vi "Canny分割算法.vi"() -> ()   [LabVIEW 2018]
uses:
  <vilib>/Utility/error.llb/DialogType.ctl
  <vilib>/vision/NI_Vision_Development_Module.lvlib
  Dll/Canny_fillhole.dll
panel:
  in  "保存":bool
  out "像素当量单位":string
  out "像素当量":string
  out "是否进行像素标定":bool
  in  "单帧回看":bool
  out "火焰帧数":string
  in  "重新选择":bool
  in  "火焰详细参数":bool
  out "叠加部分":string
  out "单帧部分":string
  out "原图":T1(plugin-control)
  in  "返回主界面":bool
  in  "程序停止":bool
  out "Progress Bar":i32(slide) max=41 scale=-1.0..41.0
  out "单帧火焰":T1(plugin-control)
  out "叠加火焰":T1(plugin-control)
  # "基于Canny算法的炮口火焰分割"
  # "火\n焰\n参\n数"
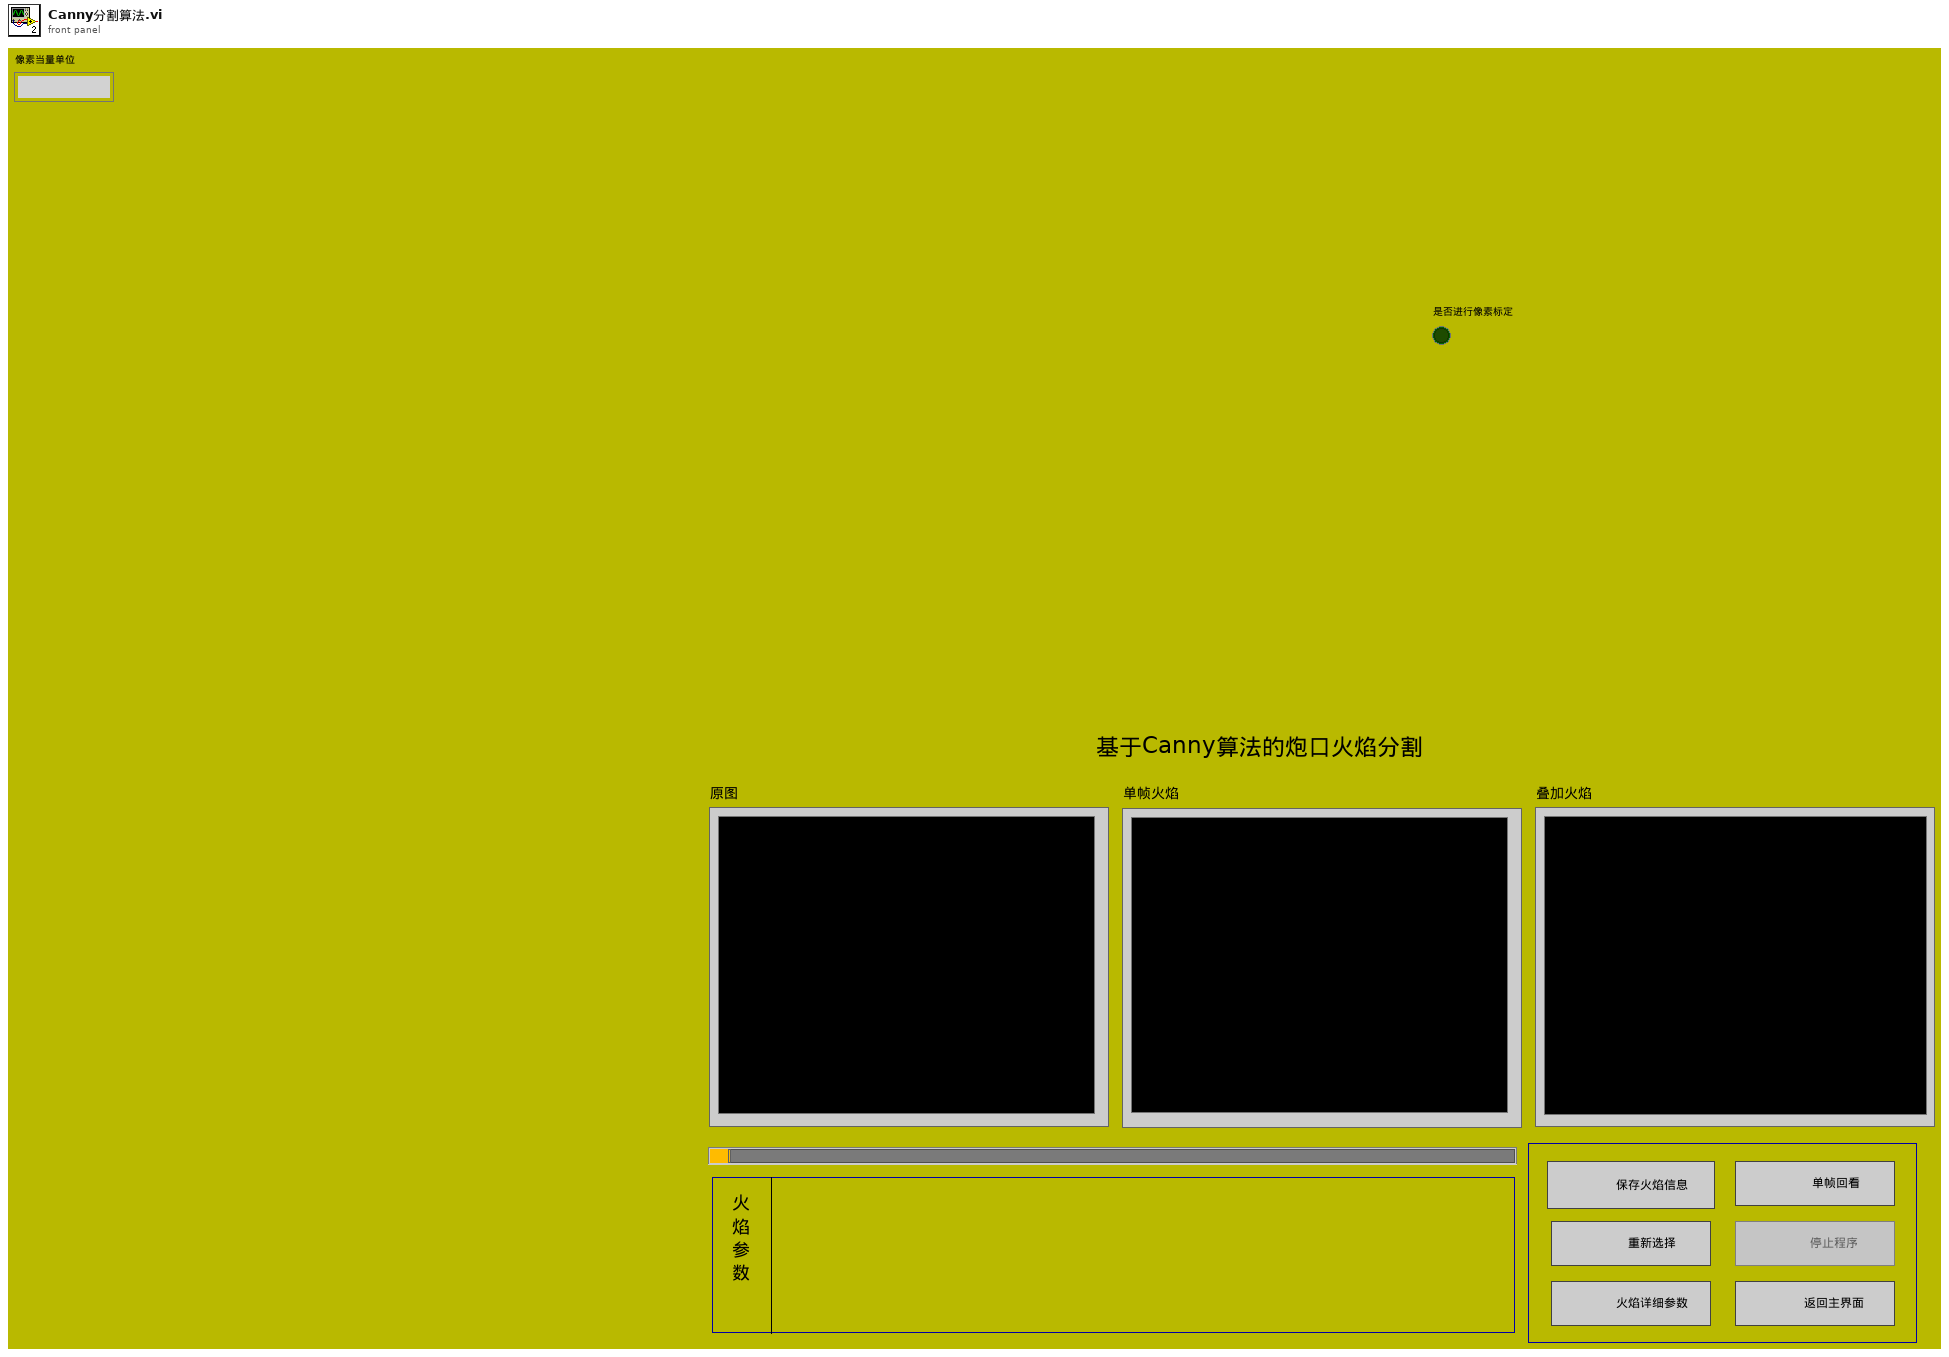
[diagram p1: front panel]
types:
  T1 = typedef "IMAQ Image.ctl" = refnum<image>
  T2 = enum8{"Enabled", "Disabled", "Disabled and Grayed Out"}
  T3 = enum32{"Invalid", "Standard", "Closed", "Hidden", "Minimized", "Maximized"}
  T4 = typedef "DialogType.ctl" = u16
  T5 = typedef "Image Type" = u32
  T6 = typedef "IMAQ AVI2 Refnum.ctl" = refnum<k20>
  T7 = cluster{"Width":u32, "Height":u32, "Frames Per Second":u32, "Codec":string, "Has Data":bool}
  T8 = typedef "ROI Descriptor" = cluster{"Global Rectangle":i32[], "Contours":cluster{"ID":enum32{"External", "Internal"}, "Type":u32, "Coordinates":i32[]}[]}
  T9 = cluster{"Area":dbl, "Number of Holes":dbl, "Bounding Rect":cluster{"Left":dbl, "Top":dbl, "Right":dbl, "Bottom":dbl}, "Center of Mass":cluster{"X":dbl, "Y":dbl}, "Orientation":dbl, "Dimensions":cluster{"Width":dbl, "Height":dbl}}[]
  T10 = cluster{"Particle Reports (Pixels)[0]":cluster{"Area":dbl, "Number of Holes":dbl, "Bounding Rect":cluster{"Left":dbl, "Top":dbl, "Right":dbl, "Bottom":dbl}, "Center of Mass":cluster{"X":dbl, "Y":dbl}, "Orientation":dbl, "Dimensions":cluster{"Width":dbl, "Height":dbl}}, "Particle Reports (Pixels)[1]":cluster{"Area":dbl, "Number of Holes":dbl, "Bounding Rect":cluster{"Left":dbl, "Top":dbl, "Right":dbl, "Bottom":dbl}, "Center of Mass":cluster{"X":dbl, "Y":dbl}, "Orientation":dbl, "Dimensions":cluster{"Width":dbl, "Height":dbl}}, "Particle Reports (Pixels)[2]":cluster{"Area":dbl, "Number of Holes":dbl, "Bounding Rect":cluster{"Left":dbl, "Top":dbl, "Right":dbl, "Bottom":dbl}, "Center of Mass":cluster{"X":dbl, "Y":dbl}, "Orientation":dbl, "Dimensions":cluster{"Width":dbl, "Height":dbl}}, "Particle Reports (Pixels)[3]":cluster{"Area":dbl, "Number of Holes":dbl, "Bounding Rect":cluster{"Left":dbl, "Top":dbl, "Right":dbl, "Bottom":dbl}, "Center of Mass":cluster{"X":dbl, "Y":dbl}, "Orientation":dbl, "Dimensions":cluster{"Width":dbl, "Height":dbl}}, "Particle Reports (Pixels)[4]":cluster{"Area":dbl, "Number of Holes":dbl, "Bounding Rect":cluster{"Left":dbl, "Top":dbl, "Right":dbl, "Bottom":dbl}, "Center of Mass":cluster{"X":dbl, "Y":dbl}, "Orientation":dbl, "Dimensions":cluster{"Width":dbl, "Height":dbl}}, "Particle Reports (Pixels)[5]":cluster{"Area":dbl, "Number of Holes":dbl, "Bounding Rect":cluster{"Left":dbl, "Top":dbl, "Right":dbl, "Bottom":dbl}, "Center of Mass":cluster{"X":dbl, "Y":dbl}, "Orientation":dbl, "Dimensions":cluster{"Width":dbl, "Height":dbl}}, "Particle Reports (Pixels)[6]":cluster{"Area":dbl, "Number of Holes":dbl, "Bounding Rect":cluster{"Left":dbl, "Top":dbl, "Right":dbl, "Bottom":dbl}, "Center of Mass":cluster{"X":dbl, "Y":dbl}, "Orientation":dbl, "Dimensions":cluster{"Width":dbl, "Height":dbl}}, "Particle Reports (Pixels)[7]":cluster{"Area":dbl, "Number of Holes":dbl, "Bounding Rect":cluster{"Left":dbl, "Top":dbl, "Right":dbl, "Bottom":dbl}, "Center of Mass":cluster{"X":dbl, "Y":dbl}, "Orientation":dbl, "Dimensions":cluster{"Width":dbl, "Height":dbl}}, "Particle Reports (Pixels)[8]":cluster{"Area":dbl, "Number of Holes":dbl, "Bounding Rect":cluster{"Left":dbl, "Top":dbl, "Right":dbl, "Bottom":dbl}, "Center of Mass":cluster{"X":dbl, "Y":dbl}, "Orientation":dbl, "Dimensions":cluster{"Width":dbl, "Height":dbl}}}
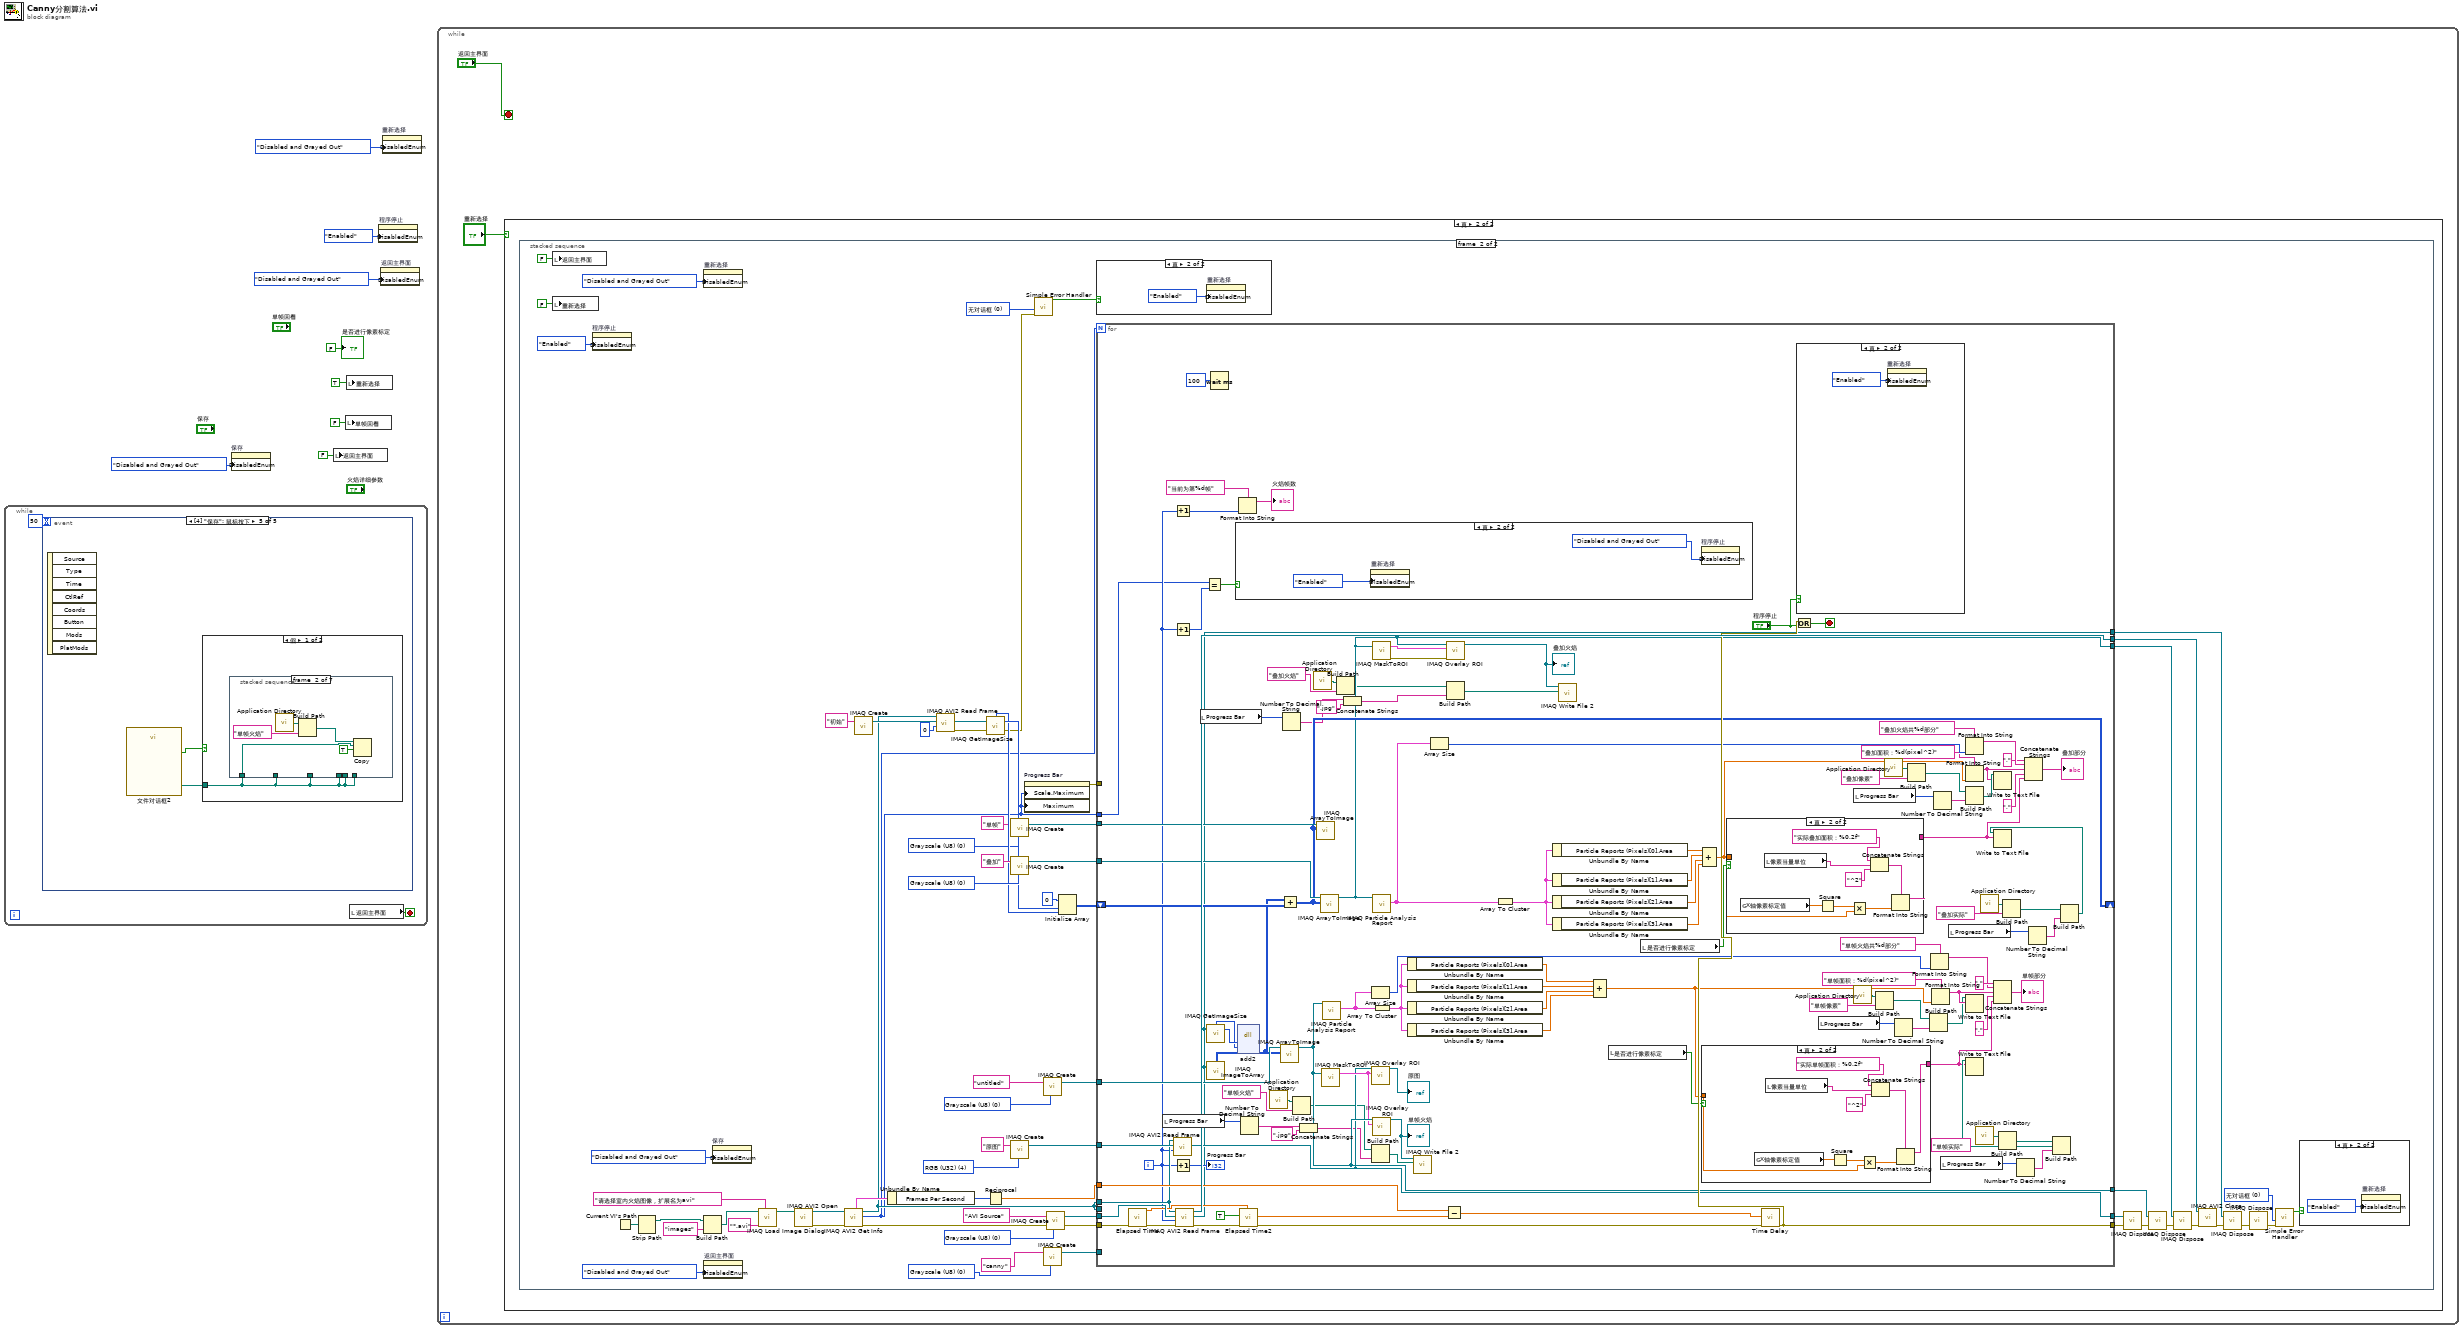
[diagram p0: block diagram]
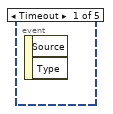
[diagram p2: hidden frame]
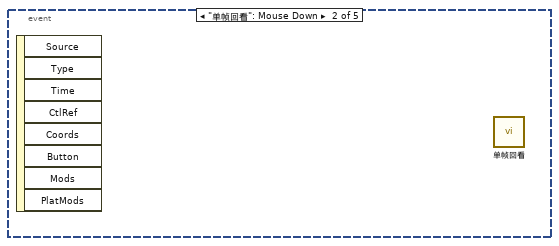
[diagram p3: hidden frame]
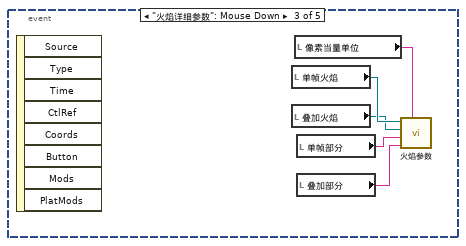
[diagram p4: hidden frame]
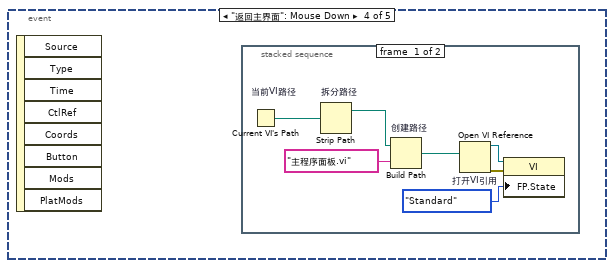
[diagram p5: hidden frame]
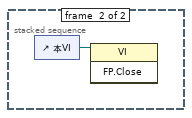
[diagram p6: hidden frame]
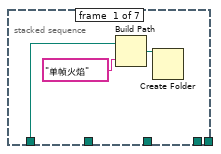
[diagram p7: hidden frame]
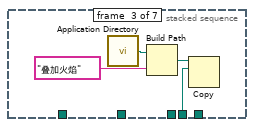
[diagram p8: hidden frame]
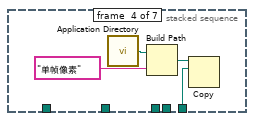
[diagram p9: hidden frame]
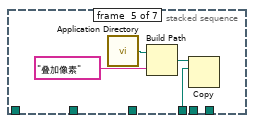
[diagram p10: hidden frame]
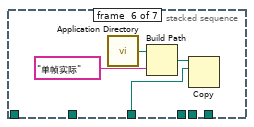
[diagram p11: hidden frame]
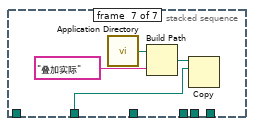
[diagram p12: hidden frame]
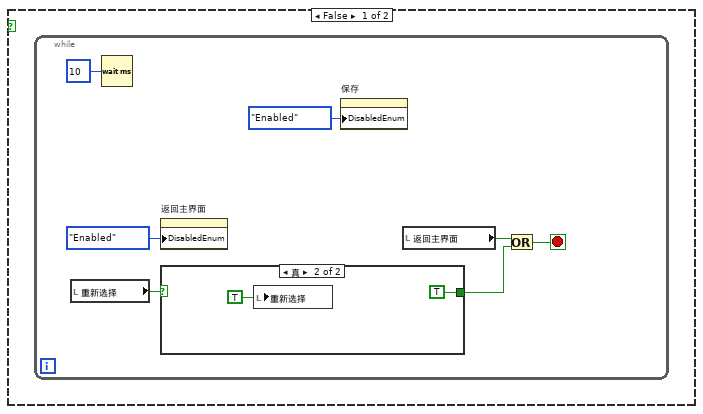
[diagram p14: hidden frame]
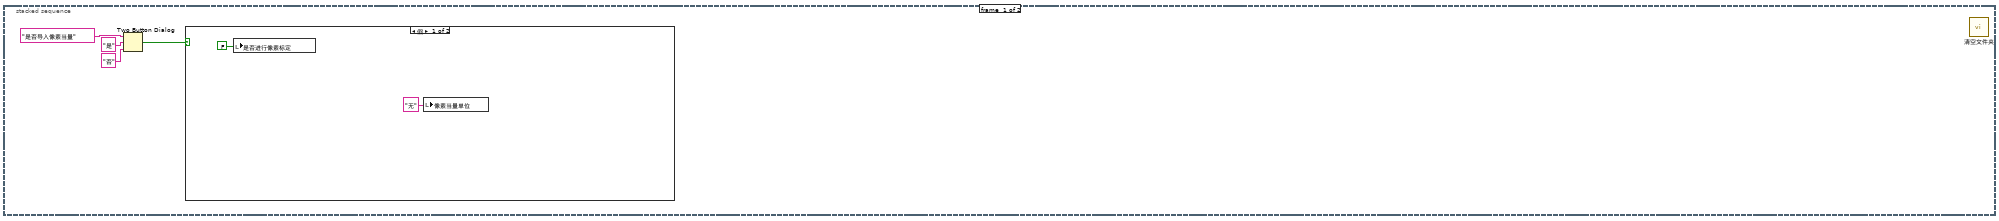
[diagram p16: hidden frame]
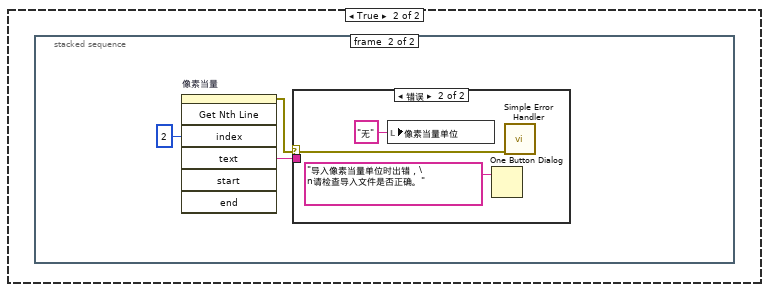
[diagram p17: hidden frame]
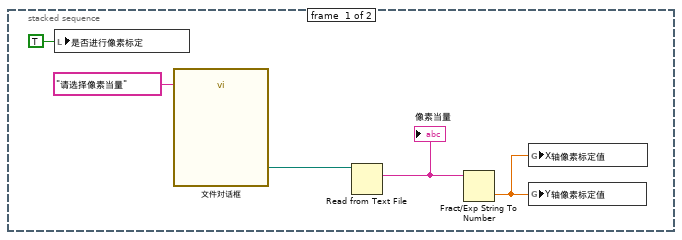
[diagram p18: hidden frame]
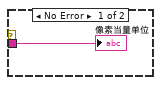
[diagram p19: hidden frame]
diagram:
  n1 = while {
    stop <- w10 stop-if-true
    n2 = event shown="[4] \"保存\": 鼠标按下" {
      selector: _ -> [_ _ _ _ _]
      dyn-events: _ -> [_ _ _ _ _]
      timeout: 50 -> [_ _ _ _ _]
      event Timeout {
        n3 = event-data() -> ()  [unwired: 1 in, 2 out]
      }
      event "单帧回看": Mouse Down {
        n4 = event-data() -> ()  [unwired: 1 in, 8 out]
        n5 = call "单帧回看.vi"() -> ()  [unwired: 28 in]
      }
      event "火焰详细参数": Mouse Down {
        n6 = event-data() -> ()  [unwired: 1 in, 8 out]
        n7 = local read "单帧火焰"() -> (w13:T1)
        n8 = local read "叠加火焰"() -> (w12:T1)
        n9 = local read "像素当量单位"() -> (w11:string)
        n10 = local read "单帧部分"() -> (w14:string)
        n11 = local read "叠加部分"() -> (w15:string)
        n12 = call "火焰参数.vi"("像素当量单位"=w11, 8:w15, 9:w14, "Image 2"=w12, "Image"=w13) -> ()  [unwired: 7 in]
      }
      event "返回主界面": Mouse Down {
        n13 = event-data() -> ()  [unwired: 1 in, 8 out]
        n14 = stacked-sequence {
          frame #0 {
            n15 = Current VI's Path "当前VI路径"() -> (path=w20:path)
            n16 = Strip Path "拆分路径"(path=w20) -> (stripped path=w22:path)  [unwired: 1 out]
            n17 = Build Path "创建路径"(base path=w22, name or relative path="主程序面板.vi" ("名称或相对路径")) -> (appended path=w21:path)
            n18 = Open VI Reference "打开VI引用"(vi path=w21) -> (vi reference=w19:refnum<vi>, error out=w18:errorcluster)  [unwired: 5 in]
            n19 = property class="VI"(reference=w19, error in=w18, "FP.State"=T3."Standard" ("前面板窗口:状态")) -> ()  [unwired: 2 out]
          }
          frame #1 {
            n20 = control-ref of="本VI"() -> (w23:refnum<vi>)
            n21 = invoke class="VI" method="FP.Close"(reference=w23) -> ()  [unwired: 2 in, 3 out]
          }
        }
      }
      event "保存": Mouse Down {
        n22 = event-data() -> ()  [unwired: 1 in, 8 out]
        n23 = call "文件对话框2"() -> ("selected path"=w25:path, "cancelled"=w24:bool)  [unwired: 12 in, 2 out]
        n24 = case shown="假" w24 {
          tunnel: w25 -> [w26 _]
          frame False {
            n25 = stacked-sequence {
              tunnel: w26 -> [w27 w31 _ _ _ _ _]
              tunnel: w26 -> [_ _ w36 _ _ _ _]
              tunnel: w26 -> [_ _ _ w40 _ _ _]
              tunnel: w26 -> [_ _ _ _ w44 _ _]
              tunnel: w26 -> [_ _ _ _ _ w48 _]
              tunnel: w26 -> [_ _ _ _ _ _ w51]
              frame #0 {
                n26 = Build Path(base path=w27, name or relative path="单帧火焰" ("名称或相对路径")) -> (appended path=w29:path)
                n27 = Create Folder(path (use dialog)=w29) -> ()  [unwired: 2 in, 3 out]
              }
              frame #1 {
                n28 = call <vilib>:"Application Directory.vi"() -> ("Application Directory"=w34:path)
                n29 = Build Path(base path=w34, name or relative path="单帧火焰" ("名称或相对路径")) -> (appended path=w32:path)
                n30 = Copy(9:TRUE ("覆盖(F)"), 10:w31, 11:w32) -> ()  [unwired: 2 in, 3 out]
              }
              frame #2 {
                n31 = call <vilib>:"Application Directory.vi"() -> ("Application Directory"=w37:path)
                n32 = Build Path(base path=w37, name or relative path="叠加火焰" ("名称或相对路径")) -> (appended path=w38:path)
                n33 = Copy(10:w36, 11:w38) -> ()  [unwired: 3 in, 3 out]
              }
              frame #3 {
                n34 = call <vilib>:"Application Directory.vi"() -> ("Application Directory"=w41:path)
                n35 = Build Path(base path=w41, name or relative path="单帧像素" ("名称或相对路径")) -> (appended path=w42:path)
                n36 = Copy(10:w40, 11:w42) -> ()  [unwired: 3 in, 3 out]
              }
              frame #4 {
                n37 = call <vilib>:"Application Directory.vi"() -> ("Application Directory"=w45:path)
                n38 = Build Path(base path=w45, name or relative path="叠加像素" ("名称或相对路径")) -> (appended path=w46:path)
                n39 = Copy(10:w44, 11:w46) -> ()  [unwired: 3 in, 3 out]
              }
              frame #5 {
                n40 = call <vilib>:"Application Directory.vi"() -> ("Application Directory"=w49:path)
                n41 = Build Path(base path=w49, name or relative path="单帧实际" ("名称或相对路径")) -> (appended path=w50:path)
                n42 = Copy(10:w48, 11:w50) -> ()  [unwired: 3 in, 3 out]
              }
              frame #6 {
                n43 = call <vilib>:"Application Directory.vi"() -> ("Application Directory"=w53:path)
                n44 = Build Path(base path=w53, name or relative path="叠加实际" ("名称或相对路径")) -> (appended path=w54:path)
                n45 = Copy(10:w51, 11:w54) -> ()  [unwired: 3 in, 3 out]
              }
            }
          }
          frame True {
          }
        }
      }
    }
    n46 = local read "返回主界面"() -> (w10:bool)
  }
  n47 = property on="保存" class="Bool (严格)"("DisabledEnum"=T2."Disabled and Grayed Out" ("禁用")) -> ()  [unwired: 2 in, 2 out]
  n48 = local write "返回主界面"(FALSE ("重新选择")) -> ()
  n49 = local write "单帧回看"(FALSE ("重新选择")) -> ()
  n50 = local write "重新选择"(TRUE ("重新选择")) -> ()
  n51 = property on="程序停止" class="Bool"("DisabledEnum"=T2."Enabled" ("禁用")) -> ()  [unwired: 2 in, 2 out]
  n52 = property on="返回主界面" class="Bool (严格)"("DisabledEnum"=T2."Disabled and Grayed Out" ("禁用")) -> ()  [unwired: 2 in, 2 out]
  n53 = property on="重新选择" class="Bool (严格)"("DisabledEnum"=T2."Disabled and Grayed Out" ("禁用")) -> ()  [unwired: 2 in, 2 out]
  n54 = while {
    stop <- "返回主界面" stop-if-true
    n55 = case shown="真" "重新选择" {
      frame False {
        n56 = while {
          stop <- w59 stop-if-true
          n57 = local read "重新选择"() -> (w62:bool)
          n58 = Wait (ms)(milliseconds to wait=u32 10 ("等待时间（毫秒）")) -> ()  [unwired: 1 out]
          n59 = property on="返回主界面" class="Bool (严格)"("DisabledEnum"=T2."Enabled" ("禁用")) -> ()  [unwired: 2 in, 2 out]
          n60 = case shown="真" w62 {
            tunnel: [_ TRUE] -> w60
            frame False {
            }
            frame True {
              n61 = local write "重新选择"(TRUE ("重新选择")) -> ()
            }
          }
          n62 = property on="保存" class="Bool (严格)"("DisabledEnum"=T2."Enabled" ("禁用")) -> ()  [unwired: 2 in, 2 out]
          n63 = local read "返回主界面"() -> (w61:bool)
          n64 = Or(x=w61, y=w60) -> (x .or. y?=w59:bool)
        }
      }
      frame True {
        n65 = stacked-sequence {
          frame #0 {
            n66 = Two Button Dialog(message="是否导入像素当量" ("消息"), 1:"否" ("F按钮名称（“取消”）"), 2:"是" ("T按钮名称（“确定”）")) -> (T button?=w69:bool)
            n67 = case shown="假" w69 {
              frame False {
                n68 = local write "是否进行像素标定"(FALSE ("是否进行像素标定")) -> ()
                n69 = local write "像素当量单位"("无" ("像素当量单位")) -> ()
              }
              frame True {
                n70 = stacked-sequence {
                  frame #0 {
                    n71 = local write "是否进行像素标定"(TRUE ("是否进行像素标定")) -> ()
                    n72 = call "文件对话框"("default name"="请选择像素当量") -> ("selected path"=w74:path)  [unwired: 11 in, 3 out]
                    n73 = Read from Text File(file (use dialog)=w74) -> (text=w75:string)  [unwired: 3 in, 3 out]
                    "像素当量" <- w75
                    n74 = Fract/Exp String To Number(string=w75) -> (number=w76:dbl)  [unwired: 3 in, 1 out]
                    n75 = global write "全局变量.vi" "X轴像素标定值"(w76) -> ()
                    n76 = global write "全局变量.vi" "Y轴像素标定值"(w76) -> ()
                  }
                  frame #1 {
                    n77 = invoke on="像素当量" class="Str" method="Get Nth Line"("index"=u32 2 ("行索引")) -> (error out=w77:errorcluster, "text"=w78:string)  [unwired: 6 in, 5 out]
                    n78 = case shown="错误" w77 {
                      selector: w77 -> [_ w83]
                      tunnel: w78 -> [w80 _]
                      frame No Error {
                        "像素当量单位" <- w80
                      }
                      frame Error {
                        n79 = local write "像素当量单位"("无" ("像素当量单位")) -> ()
                        n80 = One Button Dialog(message="导入像素当量单位时出错，\n请检查导入文件是否正确。" ("消息")) -> ()  [unwired: 1 in, 1 out]
                        n81 = call <vilib>:"Simple Error Handler.vi"("error in (no error)"=w83) -> ()  [unwired: 4 in, 5 out]
                      }
                    }
                  }
                }
              }
            }
            n82 = call "清空文件夹.vi"() -> ()  [unwired: 12 in]
          }
          frame #1 {
            w94 = T4 0 items=["无对话框", "确定信息", "继续或停止信息", "确定信息＋警告", "继续/停止+警告"] ("type of dialog (OK msg:1)")
            w95 = T4 0 items=["无对话框", "确定信息", "继续或停止信息", "确定信息＋警告", "继续/停止+警告"] ("type of dialog (OK msg:1)")
            w106 = T5 0 items=["Grayscale (U8)", "Grayscale (I16)", "Grayscale (SGL)", "Complex (CSG)", "RGB (U32)", "HSL (U32)", "RGB (U64)", "Grayscale (U16)"] ("Image Type")
            w107 = T5 4 items=["Grayscale (U8)", "Grayscale (I16)", "Grayscale (SGL)", "Complex (CSG)", "RGB (U32)", "HSL (U32)", "RGB (U64)", "Grayscale (U16)"] ("Image Type")
            w111 = T5 0 items=["Grayscale (U8)", "Grayscale (I16)", "Grayscale (SGL)", "Complex (CSG)", "RGB (U32)", "HSL (U32)", "RGB (U64)", "Grayscale (U16)"] ("Image Type")
            w132 = T5 0 items=["Grayscale (U8)", "Grayscale (I16)", "Grayscale (SGL)", "Complex (CSG)", "RGB (U32)", "HSL (U32)", "RGB (U64)", "Grayscale (U16)"] ("Image Type")
            w136 = T5 0 items=["Grayscale (U8)", "Grayscale (I16)", "Grayscale (SGL)", "Complex (CSG)", "RGB (U32)", "HSL (U32)", "RGB (U64)", "Grayscale (U16)"] ("Image Type")
            w137 = T5 0 items=["Grayscale (U8)", "Grayscale (I16)", "Grayscale (SGL)", "Complex (CSG)", "RGB (U32)", "HSL (U32)", "RGB (U64)", "Grayscale (U16)"] ("Image Type")
            n83 = local write "返回主界面"(FALSE ("重新选择")) -> ()
            n84 = local write "重新选择"(FALSE ("重新选择")) -> ()
            n85 = property on="程序停止" class="Bool"("DisabledEnum"=T2."Enabled" ("禁用")) -> ()  [unwired: 2 in, 2 out]
            n86 = Current VI's Path() -> (path=w90:path)
            n87 = Strip Path(path=w90) -> (stripped path=w91:path)  [unwired: 1 out]
            n88 = property on="重新选择" class="Bool (严格)"("DisabledEnum"=T2."Disabled and Grayed Out" ("禁用")) -> ()  [unwired: 2 in, 2 out]
            n89 = Build Path(base path=w91, name or relative path="images") -> (appended path=w88:path)
            n90 = property on="返回主界面" class="Bool (严格)"("DisabledEnum"=T2."Disabled and Grayed Out" ("禁用")) -> ()  [unwired: 2 in, 2 out]
            n91 = property on="保存" class="Bool (严格)"("DisabledEnum"=T2."Disabled and Grayed Out" ("禁用")) -> ()  [unwired: 2 in, 2 out]
            n92 = call "IMAQ Load Image Dialog"("Prompt"="请选择室内火焰图像，扩展名为avi" ("prompt"), "Pattern"="*.avi", "Start Path"=w88) -> ("Path"=w119:path)  [unwired: 6 in, 2 out]
            n93 = call "IMAQ AVI2 Open"("AVI File Path"=w119) -> ("error out"=w148:errorcluster, "AVI Refnum"=w147:T6)  [unwired: 2 in, 7 out]
            n94 = call "IMAQ AVI2 Get Info"("error in (no error)"=w148, "AVI Refnum"=w147) -> ("error out"=w145:errorcluster, "Number of Frames"=w98:u32, "AVI Refnum (duplicate)"=w123:T6, "Frame Data"=w149:T7)  [unwired: 6 out]
            n95 = call "IMAQ Create"("Image Name"="初始") -> ("New Image"=w129:T1)  [unwired: 4 in, 1 out]
            n96 = Unbundle By Name(w149) -> ("Frames Per Second"=w140:u32)
            n97 = call "IMAQ AVI2 Read Frame"("Frame Number"=u32 0, "Image"=w129, "AVI Refnum"=w123) -> ("error out"=w97:errorcluster, "Image Out"=w127:T1)  [unwired: 1 in, 6 out]
            n98 = call "IMAQ GetImageSize"("Image"=w127, "error in (no error)"=w97) -> ("Y Resolution"=w126:i32, "X Resolution"=w122:i32, "error out"=w96:errorcluster)  [unwired: 2 in]
            n99 = Reciprocal(x=w140) -> (1/x=w139:dbl)
            n100 = call "IMAQ Create"("Image Name"="单帧", "Image Type"=w111) -> ("New Image"=w113:T1)  [unwired: 3 in, 1 out]
            n101 = call "IMAQ Create"("Image Name"="叠加", "Image Type"=w132) -> ("New Image"=w131:T1)  [unwired: 3 in, 1 out]
            n102 = call "IMAQ Create"("Image Name"="原图", "Image Type"=w107) -> ("New Image"=w109:T1)  [unwired: 2 in, 2 out]
            n103 = property on="Progress Bar" class="Slide (严格)"("Scale.Maximum"=w98, "Maximum"=w98) -> (error out=w138:errorcluster)  [unwired: 2 in, 1 out]
            n104 = call <vilib>:"Simple Error Handler.vi"("type of dialog (OK msg:1)"=w95, "error in (no error)"=w96) -> ("error?"=w92:bool)  [unwired: 3 in, 4 out]
            n105 = call "IMAQ Create"("Image Name"="untitled", "Image Type"=w136) -> ("New Image"=w135:T1)  [unwired: 2 in, 2 out]
            n106 = call "IMAQ Create"("Image Name"="canny", "Image Type"=w106) -> ("New Image"=w104:T1)  [unwired: 2 in, 2 out]
            n107 = call "IMAQ Create"("Image Name"="AVI Source", "Image Type"=w137, "error in (no error)"=w145) -> ("New Image"=w143:T1, "error out"=w144:errorcluster)  [unwired: 1 in, 1 out]
            n108 = Initialize Array(u8 0 ("元素"), w126, w122) -> (w124:u8[][])
            n109 = case shown="真" w92 {
              frame False {
              }
              frame True {
                n110 = property on="重新选择" class="Bool (严格)"("DisabledEnum"=T2."Enabled" ("禁用")) -> ()  [unwired: 2 in, 2 out]
              }
            }
            n111 = for {
              N: w98 -> [_]
              tunnel: w143 -> [w270]
              tunnel: [w269] -> w146
              tunnel: [w260] -> w103
              tunnel: w144 -> [w268]
              tunnel: w123 -> [w247]
              tunnel: [w219] -> w141
              tunnel: w139 -> [w266]
              tunnel: w138 -> [_]
              tunnel: w135 -> [w251]
              tunnel: w131 -> [w257]
              shift-right: [w250] -> _
              shift-left: w124 -> [w256]
              tunnel: w123 -> [_]
              tunnel: [w232] -> w118
              tunnel: w113 -> [w252]
              tunnel: [w235] -> w110
              tunnel: w109 -> [w248]
              tunnel: w104 -> [_]
              tunnel: [w220] -> w101
              tunnel: w98 -> [w222]
              i -> [w223]
              stop <- w259 stop-if-true
              n112 = call "Elapsed Time"("error in (no error)"=w268) -> ("Present (s)"=w264:dbl, "error out"=w267:errorcluster)  [unwired: 11 in, 6 out]
              n113 = local read "Progress Bar"() -> (w209:i32)
              n114 = call "IMAQ AVI2 Read Frame"("Frame Number"=w223, "Image"=w248, "AVI Refnum"=w247) -> ("Image Out"=w220:T1)  [unwired: 1 in, 7 out]
              n115 = Increment(x=w223) -> (x+1=w227:i32)
              n116 = Increment(x=w223) -> (x+1=w221:i32)
              n117 = Increment(x=w223) -> (x+1=→"Progress Bar":i32)
              n118 = call "IMAQ AVI2 Read Frame"("error in (no error)"=w267, "Frame Number"=w223, "Image"=w270, "AVI Refnum"=w247) -> ("error out"=w262:errorcluster, "Image Out"=w219:T1, "AVI Refnum (duplicate)"=w269:T6)  [unwired: 5 out]
              n119 = local read "Progress Bar"() -> (w204:i32)
              n120 = Equal?(x=w222, y=w221) -> (x = y?=w224:bool)
              n121 = call "IMAQ GetImageSize"("Image"=w219) -> ("Y Resolution"=w255:i32, "X Resolution"=w254:i32)  [unwired: 3 in, 1 out]
              n122 = call "IMAQ ImageToArray"("Image"=w219) -> ("Image Pixels (U8)"=w253:u8[][])  [unwired: 3 in, 4 out]
              n123 = Wait (ms)(milliseconds to wait=u32 100 ("等待时间（毫秒）")) -> ()  [unwired: 1 out]
              n124 = case shown="真" w224 {
                frame False {
                }
                frame True {
                  n125 = property on="重新选择" class="Bool (严格)"("DisabledEnum"=T2."Enabled" ("禁用")) -> ()  [unwired: 2 in, 2 out]
                  n126 = property on="程序停止" class="Bool"("DisabledEnum"=T2."Disabled and Grayed Out" ("禁用")) -> ()  [unwired: 2 in, 2 out]
                }
              }
              n127 = dll-call lib="PTH2Fabs DsdhProgramme_GuShiJu火焰分割DllCanny_fillhole.dll" fn="add2"("rows"=w255, "cols"=w254, "data"=w253) -> ("data"=w249:u8[][])  [unwired: 6 in, 2 out]
              n128 = Format Into String(format string="当前为第%d帧" ("格式字符串"), w227) -> (resulting string=→"火焰帧数":string)  [unwired: 2 in, 1 out]
              n129 = call "Elapsed Time2"("Reset"=TRUE, "error in (no error)"=w262, "Set Start Time (s)"=w264) -> ("Elapsed Time (s)"=w261:dbl, "error out"=w229:errorcluster)  [unwired: 9 in, 6 out]
              n130 = Number To Decimal String(number=w209) -> (decimal integer string=w208:string)  [unwired: 1 in]
              n131 = call <vilib>:"Application Directory.vi"() -> ("Application Directory"=w215:path)
              n132 = call "IMAQ ArrayToImage"("Image Pixels (U8)"=w249, "Image"=w251) -> ("Image Out"=w235:T1)  [unwired: 8 in, 1 out]
              n133 = Add(x=w249, y=w256) -> (x+y=w250:u8[][])
              n134 = Number To Decimal String(number=w204) -> (decimal integer string=w205:string)  [unwired: 1 in]
              n135 = Build Path(base path=w215, name or relative path="单帧火焰" ("名称或相对路径")) -> (appended path=w213:path)
              n136 = Concatenate Strings(w208, ".jpg" ("字符串")) -> (w212:string)
              n137 = call <vilib>:"Application Directory.vi"() -> ("Application Directory"=w199:path)
              n138 = call "IMAQ ArrayToImage"("Image Pixels (U8)"=w250, "Image"=w252) -> ()  [unwired: 8 in, 2 out]
              n139 = call "IMAQ ArrayToImage"("Image Pixels (U8)"=w250, "Image"=w257) -> ("Image Out"=w232:T1)  [unwired: 8 in, 1 out]
              n140 = call "IMAQ MaskToROI"("Image"=w235) -> ("ROI Descriptor"=w230:T8)  [unwired: 6 in, 2 out]
              n141 = call "IMAQ Particle Analysis Report"("Image"=w235) -> ("Particle Reports (Pixels)"=w237:T9)  [unwired: 5 in, 5 out]
              n142 = Build Path(base path=w199, name or relative path="叠加火焰" ("名称或相对路径")) -> (appended path=w201:path)
              n143 = Concatenate Strings(w205, ".jpg" ("字符串")) -> (w202:string)
              n144 = Array Size(array=w237) -> (size(s)=w238:i32)
              n145 = call "IMAQ Overlay ROI"("ROI Descriptor"=w230, "Image"=w220) -> ("Image Out"=→"原图":T1)  [unwired: 8 in, 1 out]
              n146 = Build Path(base path=w213, name or relative path=w212) -> (appended path=w207:path)
              n147 = call "IMAQ Overlay ROI"("ROI Descriptor"=w230, "Image"=w235) -> ("Image Out"=w210:T1)  [unwired: 8 in, 1 out]
              "单帧火焰" <- w210
              n148 = call "IMAQ MaskToROI"("Image"=w232) -> ("ROI Descriptor"=w233:T8, "error out"=w234:errorcluster)  [unwired: 6 in, 1 out]
              n149 = call "IMAQ Particle Analysis Report"("Image"=w232) -> ("Particle Reports (Pixels)"=w236:T9)  [unwired: 5 in, 5 out]
              n150 = Array To Cluster(array=w237) -> (cluster=w217:T10)
              n151 = Unbundle By Name(w217) -> ("Particle Reports (Pixels)[0].Area"=w246:dbl)
              n152 = Unbundle By Name(w217) -> ("Particle Reports (Pixels)[1].Area"=w245:dbl)
              n153 = Unbundle By Name(w217) -> ("Particle Reports (Pixels)[2].Area"=w244:dbl)
              n154 = Unbundle By Name(w217) -> ("Particle Reports (Pixels)[3].Area"=w243:dbl)
              n155 = call-poly "IMAQ Write File 2"("File Path"=w207, "Image"=w210) -> ()  [unwired: 8 in, 2 out]
              n156 = Array Size(array=w236) -> (size(s)=w185:i32)
              n157 = Subtract(x=w266, y=w261) -> (x-y=w265:dbl)
              n158 = call "IMAQ Overlay ROI"("error in (no error)"=w234, "ROI Descriptor"=w233, "Image"=w232) -> ("Image Out"=w198:T1)  [unwired: 7 in, 1 out]
              "叠加火焰" <- w198
              n159 = Build Path(base path=w201, name or relative path=w202) -> (appended path=w206:path)
              n160 = Array To Cluster(array=w236) -> (cluster=w218:T10)
              n161 = Unbundle By Name(w218) -> ("Particle Reports (Pixels)[0].Area"=w242:dbl)
              n162 = Unbundle By Name(w218) -> ("Particle Reports (Pixels)[1].Area"=w241:dbl)
              n163 = Unbundle By Name(w218) -> ("Particle Reports (Pixels)[2].Area"=w240:dbl)
              n164 = Unbundle By Name(w218) -> ("Particle Reports (Pixels)[3].Area"=w216:dbl)
              n165 = call-poly "IMAQ Write File 2"("File Path"=w206, "Image"=w198) -> ()  [unwired: 8 in, 2 out]
              n166 = Compound Arithmetic op=ADD(w246, w245, w244, w243) -> (w192:dbl)
              n167 = local read "是否进行像素标定"() -> (w195:bool)
              n168 = local read "是否进行像素标定"() -> (w189:bool)
              n169 = case shown="真" w195 {
                tunnel: ["未进行像素标定" ("初始字符串") w286] -> w171
                tunnel: w192 -> [_ w288]
                frame False {
                }
                frame True {
                  n170 = global read "全局变量.vi" "X轴像素标定值"() -> (w290:dbl)
                  n171 = local read "像素当量单位"() -> (w283:string)
                  n172 = Square(x=w290) -> (x^2=w289:dbl)
                  n173 = Multiply(x=w289, y=w288) -> (x*y=w287:dbl)
                  n174 = Concatenate Strings("实际单帧面积：%0.2f" ("初始字符串"), w283, "^2" ("字符串")) -> (w282:string)
                  n175 = Format Into String(format string=w282, w287) -> (resulting string=w286:string)  [unwired: 2 in, 1 out]
                }
              }
              n176 = Compound Arithmetic op=ADD(w242, w241, w240, w216) -> (w184:dbl)
              n177 = case shown="真" w189 {
                tunnel: ["未进行像素标定" ("初始字符串") w277] -> w157
                tunnel: w184 -> [_ w276]
                frame False {
                }
                frame True {
                  n178 = global read "全局变量.vi" "X轴像素标定值"() -> (w280:dbl)
                  n179 = local read "像素当量单位"() -> (w275:string)
                  n180 = Square(x=w280) -> (x^2=w279:dbl)
                  n181 = Multiply(x=w279, y=w276) -> (x*y=w278:dbl)
                  n182 = Concatenate Strings("实际叠加面积：%0.2f" ("初始字符串"), w275, "^2" ("字符串")) -> (w272:string)
                  n183 = Format Into String(format string=w272, w278) -> (resulting string=w277:string)  [unwired: 2 in, 1 out]
                }
              }
              n184 = call "Time Delay"("error in (no error)"=w229, "Delay Time (s)"=w265) -> ("error out"=w260:errorcluster)  [unwired: 9 in]
              n185 = Or(x=w260, y="程序停止") -> (x .or. y?=w259:bool)
              n186 = case shown="真" "程序停止" {
                frame False {
                }
                frame True {
                  n187 = property on="重新选择" class="Bool (严格)"("DisabledEnum"=T2."Enabled" ("禁用")) -> ()  [unwired: 2 in, 2 out]
                }
              }
              n188 = local read "Progress Bar"() -> (w180:i32)
              n189 = call <vilib>:"Application Directory.vi"() -> ("Application Directory"=w183:path)
              n190 = local read "Progress Bar"() -> (w164:i32)
              n191 = Build Path(base path=w183, name or relative path="单帧像素" ("名称或相对路径")) -> (appended path=w181:path)
              n192 = call <vilib>:"Application Directory.vi"() -> ("Application Directory"=w161:path)
              n193 = Number To Decimal String(number=w180) -> (decimal integer string=w179:string)  [unwired: 1 in]
              n194 = Build Path(base path=w161, name or relative path="叠加像素" ("名称或相对路径")) -> (appended path=w163:path)
              n195 = Build Path(base path=w181, name or relative path=w179) -> (appended path=w177:path)
              n196 = Format Into String(format string="单帧火焰共%d部分" ("初始字符串"), w238) -> (resulting string=w196:string)  [unwired: 2 in, 1 out]
              n197 = Format Into String(format string="单帧面积：%d(pixel^2)" ("初始字符串"), w192) -> (resulting string=w178:string)  [unwired: 2 in, 1 out]
              n198 = Number To Decimal String(number=w164) -> (decimal integer string=w160:string)  [unwired: 1 in]
              n199 = local read "Progress Bar"() -> (w175:i32)
              n200 = local read "Progress Bar"() -> (w165:i32)
              n201 = Format Into String(format string="叠加火焰共%d部分" ("初始字符串"), w185) -> (resulting string=w188:string)  [unwired: 2 in, 1 out]
              n202 = Format Into String(format string="叠加面积：%d(pixel^2)" ("初始字符串"), w184) -> (resulting string=w158:string)  [unwired: 2 in, 1 out]
              n203 = Build Path(base path=w163, name or relative path=w160) -> (appended path=w159:path)
              n204 = Write to Text File(file (use dialog)=w177, text=w178) -> ()  [unwired: 2 in, 3 out]
              n205 = call <vilib>:"Application Directory.vi"() -> ("Application Directory"=w172:path)
              n206 = call <vilib>:"Application Directory.vi"() -> ("Application Directory"=w168:path)
              n207 = Write to Text File(file (use dialog)=w159, text=w158) -> ()  [unwired: 2 in, 3 out]
              n208 = Concatenate Strings(w196, "," ("字符串"), w178, "," ("字符串"), w171) -> (→"单帧部分":string)
              n209 = Build Path(base path=w172, name or relative path="单帧实际" ("名称或相对路径")) -> (appended path=w174:path)
              n210 = Build Path(base path=w168, name or relative path="叠加实际" ("名称或相对路径")) -> (appended path=w166:path)
              n211 = Number To Decimal String(number=w175) -> (decimal integer string=w170:string)  [unwired: 1 in]
              n212 = Concatenate Strings(w188, "," ("字符串"), w158, "," ("字符串"), w157) -> (→"叠加部分":string)
              n213 = Number To Decimal String(number=w165) -> (decimal integer string=w169:string)  [unwired: 1 in]
              n214 = Build Path(base path=w174, name or relative path=w170) -> (appended path=w176:path)
              n215 = Write to Text File(file (use dialog)=w176, text=w171) -> ()  [unwired: 2 in, 3 out]
              n216 = Build Path(base path=w166, name or relative path=w169) -> (appended path=w156:path)
              n217 = Write to Text File(file (use dialog)=w156, text=w157) -> ()  [unwired: 2 in, 3 out]
            }
            n218 = call "IMAQ Dispose"("Image"=w101, "error in (no error)"=w103) -> ("error out"=w102:errorcluster)  [unwired: 1 in, 3 out]
            n219 = call "IMAQ Dispose"("Image"=w110, "error in (no error)"=w102) -> ("error out"=w117:errorcluster)  [unwired: 1 in, 3 out]
            n220 = call "IMAQ Dispose"("Image"=w118, "error in (no error)"=w117) -> ("error out"=w116:errorcluster)  [unwired: 1 in, 3 out]
            n221 = call "IMAQ AVI2 Close"("error in (no error)"=w116, "AVI Refnum"=w146) -> ("error out"=w142:errorcluster)  [unwired: 9 out]
            n222 = call "IMAQ Dispose"("Image"=w141, "error in (no error)"=w142) -> ("error out"=w115:errorcluster)  [unwired: 1 in, 3 out]
            n223 = call "IMAQ Dispose"("error in (no error)"=w115) -> ("error out"=w114:errorcluster)  [unwired: 2 in, 3 out]
            n224 = call <vilib>:"Simple Error Handler.vi"("type of dialog (OK msg:1)"=w94, "error in (no error)"=w114) -> ("error?"=w93:bool)  [unwired: 3 in, 4 out]
            n225 = case shown="真" w93 {
              frame False {
              }
              frame True {
                n226 = property on="重新选择" class="Bool (严格)"("DisabledEnum"=T2."Enabled" ("禁用")) -> ()  [unwired: 2 in, 2 out]
              }
            }
          }
        }
      }
    }
  }
  "是否进行像素标定" <- FALSE ("是否进行像素标定")
